vi "Define DataGrid Columns.vi"(8 "error in (no error)":errorcluster, 10 "ColumnSetup":T1[](array[typedef]) {"MinWidth" min=2 step=1; "AutoSizeMode" items=["None"=1, "ColumnHeader"=2, "AllCellsExceptHeader"=4, "AllCells"=6, "DisplayedCellsExceptHeader"=8, "DisplayedCells"=10, "Fill"=16]; "FillWeight" min=1 max=100}, 11 "DataGrid in":refnum<class "DataGridView.lvclass">) -> (0 "error out":errorcluster, 2 "ColumnDefs":refnum<class "GridColumn.lvclass">[](array[class]), 3 "DataGrid out":refnum<class "DataGridView.lvclass">)   [LabVIEW 2016, in "DataGrid.lvlib" / "DataGridView.lvclass"]
doc: "Defines the columns of the dataTable that is used to store all display data. If called more than once, it will add columns to the existing dataTable, so resulting in more (possibly duplicate) columns."
uses:
  <userlib>/LabVIEWdotNetDataGrid/source/DataGridView/DataGridView.lvclass
  <userlib>/LabVIEWdotNetDataGrid/source/GridColumn/ColumnDefinition.ctl
  <userlib>/LabVIEWdotNetDataGrid/source/GridColumn/ColumnType.ctl
  <userlib>/LabVIEWdotNetDataGrid/source/GridColumn/GridColumn.lvclass
  <userlib>/LabVIEWdotNetDataGrid/source/DataGridView/DataGridView.lvclass/DataGridView.ctl
  System.Windows.Forms
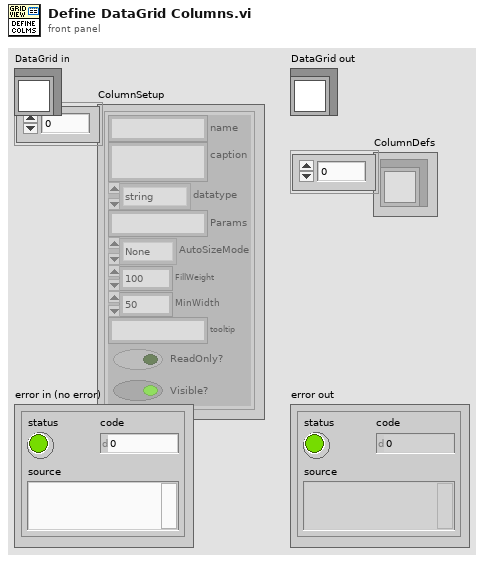
[diagram p1: front panel]
types:
  T1 = typedef "DataGrid.lvlib/GridColumn.lvclass/ColumnDefinition.ctl" = cluster{"name":string, "caption":string, "datatype":T2, "Params":string, "AutoSizeMode":i32, "FillWeight":sgl, "MinWidth":u32, "tooltip":string, "ReadOnly?":bool, "Visible?":bool}
  T2 = typedef "DataGrid.lvlib/GridColumn.lvclass/ColumnType.ctl" = enum16{"string", "image", "check", "numeric", "timestamp", "button", "combo", "link"}
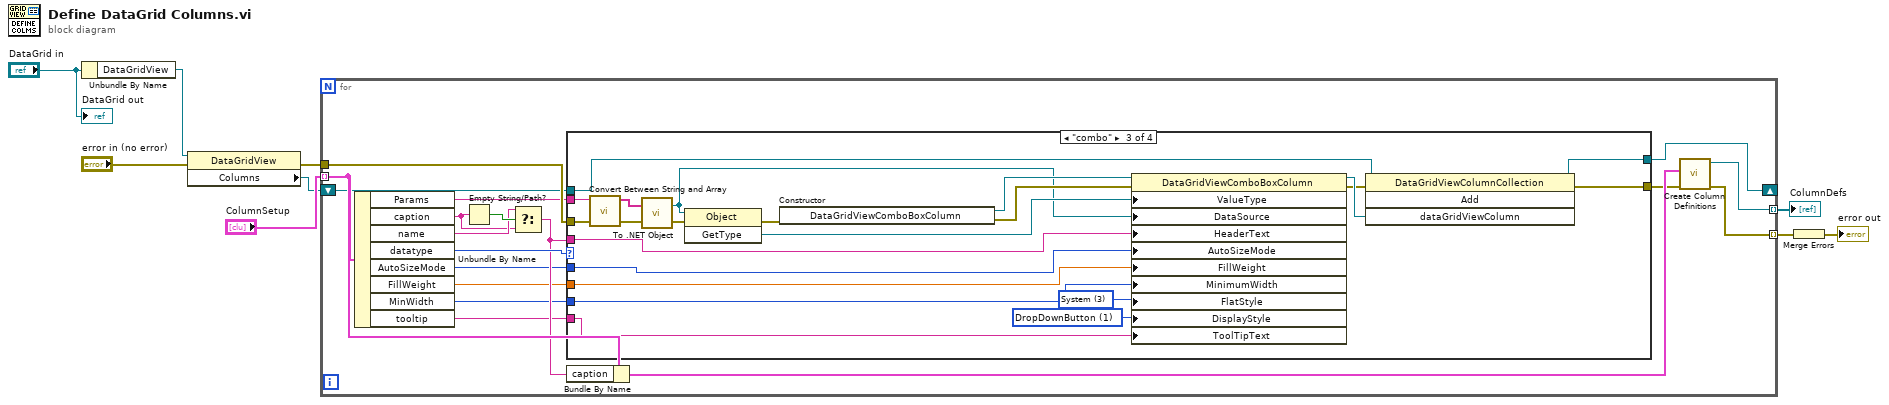
[diagram p0: block diagram]
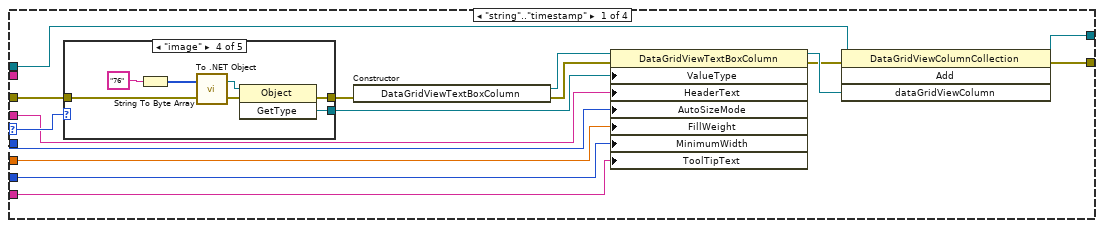
[diagram p2: hidden frame]
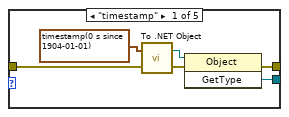
[diagram p3: hidden frame]
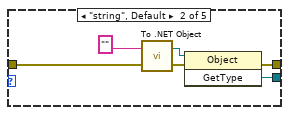
[diagram p4: hidden frame]
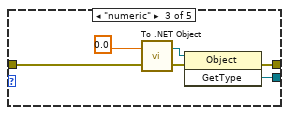
[diagram p5: hidden frame]
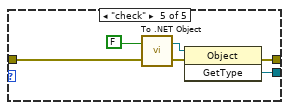
[diagram p6: hidden frame]
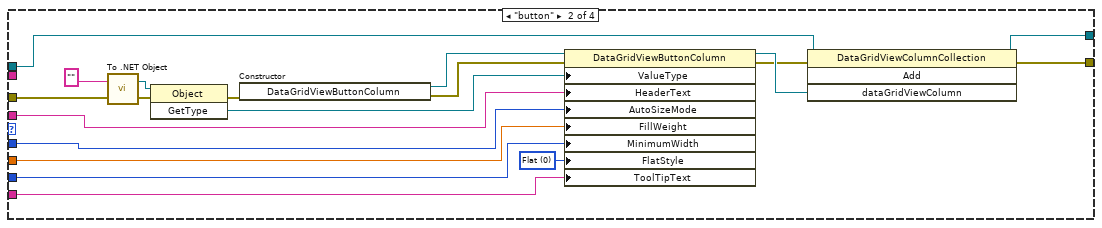
[diagram p7: hidden frame]
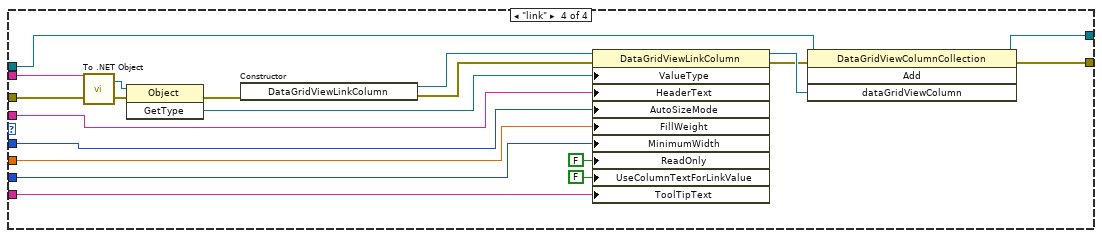
[diagram p8: hidden frame]
diagram:
  n1 = Unbundle By Name("DataGrid in") -> ("DataGridView"=w4:refnum<k24>)
  n2 = property class="DataGridView"(reference=w4, error in="error in (no error)") -> (error out=w2:errorcluster, "Columns"=w5:refnum<k24>)  [unwired: 1 out]
  n3 = for {
    tunnel: "ColumnSetup" -> [w22] mode=indexing
    tunnel: [w12] -> w7 mode=indexing
    shift-right: [w13] -> _
    shift-left: w5 -> [w14]
    tunnel: [w26] -> w6 mode=indexing
    tunnel: w2 -> [w25]
    n4 = Unbundle By Name(w22) -> ("Params"=w11:string, "caption"=w20:string, "name"=w23:string, "datatype"=w27:T2, "AutoSizeMode"=w16:i32, "FillWeight"=w17:sgl, "MinWidth"=w18:u32, "tooltip"=w10:string)
    n5 = Empty String/Path?(string/path=w20) -> (empty?=w24:bool)
    n6 = Select(t=w23, s=w24, f=w20) -> (s? t:f=w19:string)
    n7 = case shown="\"combo\"" w27 {
      selector: w27 -> [w35 _ _ _]
      tunnel: [w32 w79 w103 w122] -> w15
      tunnel: w25 -> [w43 w93 w114 w134]
      tunnel: w19 -> [w30 w76 w100 w119]
      tunnel: w18 -> [w42 w92 w113 w133]
      tunnel: w17 -> [w41 w91 w112 w132]
      tunnel: w16 -> [w40 w90 w111 w131]
      tunnel: w14 -> [w29 w78 w102 w121]
      tunnel: [w31 w77 w101 w120] -> w13
      tunnel: w11 -> [_ _ w99 w116]
      tunnel: w10 -> [w28 w75 w94 w115]
      frame "string".."timestamp" {
        n8 = case shown="\"image\"" w35 {
          tunnel: w43 -> [w47 w53 w59 w66 w72]
          tunnel: [w46 w52 w58 w65 w71] -> w38
          tunnel: [w45 w51 w57 w64 w70] -> w36
          frame "timestamp" {
            n9 = call <vilib>:"To .NET Object.vi"("error in (no error)"=w47, "anything"=timestamp(0 s since 1904-01-01) ("name")) -> ("error out"=w48:errorcluster, ".NET object"=w49:refnum<k24>)
            n10 = invoke class="Object" method="GetType"(reference=w49, error in=w48) -> (error out=w45:errorcluster, "GetType"=w46:refnum<k24>)  [unwired: 1 in, 1 out]
          }
          frame "string", Default {
            n11 = call <vilib>:"To .NET Object.vi"("error in (no error)"=w53, "anything"="") -> ("error out"=w54:errorcluster, ".NET object"=w55:refnum<k24>)
            n12 = invoke class="Object" method="GetType"(reference=w55, error in=w54) -> (error out=w51:errorcluster, "GetType"=w52:refnum<k24>)  [unwired: 1 in, 1 out]
          }
          frame "numeric" {
            n13 = call <vilib>:"To .NET Object.vi"("error in (no error)"=w59, "anything"=0.0) -> ("error out"=w60:errorcluster, ".NET object"=w61:refnum<k24>)
            n14 = invoke class="Object" method="GetType"(reference=w61, error in=w60) -> (error out=w57:errorcluster, "GetType"=w58:refnum<k24>)  [unwired: 1 in, 1 out]
          }
          frame "image" {
            n15 = String To Byte Array(string="76") -> (unsigned byte array=w62:u8[])
            n16 = call <vilib>:"To .NET Object.vi"("error in (no error)"=w66, "anything"=w62) -> ("error out"=w67:errorcluster, ".NET object"=w68:refnum<k24>)
            n17 = invoke class="Object" method="GetType"(reference=w68, error in=w67) -> (error out=w64:errorcluster, "GetType"=w65:refnum<k24>)  [unwired: 1 in, 1 out]
          }
          frame "check" {
            n18 = call <vilib>:"To .NET Object.vi"("error in (no error)"=w72, "anything"=FALSE) -> ("error out"=w73:errorcluster, ".NET object"=w74:refnum<k24>)
            n19 = invoke class="Object" method="GetType"(reference=w74, error in=w73) -> (error out=w70:errorcluster, "GetType"=w71:refnum<k24>)  [unwired: 1 in, 1 out]
          }
        }
        n20 = constructor class="DataGridViewTextBoxColumn"(error in=w36) -> (reference out=w39:refnum<k24>, error out=w37:errorcluster)  [unwired: 2 in, 1 out]
        n21 = property class="DataGridViewTextBoxColumn"(reference=w39, error in=w37, "ValueType"=w38, "HeaderText"=w30, "AutoSizeMode"=w40, "FillWeight"=w41, "MinimumWidth"=w42, "ToolTipText"=w28) -> (reference out=w34:refnum<k24>, error out=w33:errorcluster)
        n22 = invoke class="DataGridViewColumnCollection" method="Add"(reference=w29, error in=w33, "dataGridViewColumn"=w34) -> (reference out=w31:refnum<k24>, error out=w32:errorcluster)  [unwired: 1 in, 2 out]
      }
      frame "button" {
        w82 = 0 items=["Flat", "Popup", "Standard", "System"] ("FlatStyle")
        n23 = call <vilib>:"To .NET Object.vi"("error in (no error)"=w93, "anything"="") -> ("error out"=w85:errorcluster, ".NET object"=w86:refnum<k24>)
        n24 = invoke class="Object" method="GetType"(reference=w86, error in=w85) -> (error out=w88:errorcluster, "GetType"=w89:refnum<k24>)  [unwired: 1 in, 1 out]
        n25 = constructor class="DataGridViewButtonColumn"(error in=w88) -> (reference out=w83:refnum<k24>, error out=w87:errorcluster)  [unwired: 2 in, 1 out]
        n26 = property class="DataGridViewButtonColumn"(reference=w83, error in=w87, "ValueType"=w89, "HeaderText"=w76, "AutoSizeMode"=w90, "FillWeight"=w91, "MinimumWidth"=w92, "FlatStyle"=w82, "ToolTipText"=w75) -> (reference out=w81:refnum<k24>, error out=w80:errorcluster)
        n27 = invoke class="DataGridViewColumnCollection" method="Add"(reference=w78, error in=w80, "dataGridViewColumn"=w81) -> (reference out=w77:refnum<k24>, error out=w79:errorcluster)  [unwired: 1 in, 2 out]
      }
      frame "combo" {
        w97 = 1 items=["ComboBox", "DropDownButton", "Nothing"] ("DisplayStyle")
        w106 = 3 items=["Flat", "Popup", "Standard", "System"] ("FlatStyle")
        n28 = call <userlib>:"Convert Between String and Array.vi"("String"=w99) -> ("String Array"=w98:string[])  [unwired: 9 in, 1 out]
        n29 = call <vilib>:"To .NET Object.vi"("error in (no error)"=w114, "anything"=w98) -> ("error out"=w108:errorcluster, ".NET object"=w95:refnum<k24>)
        n30 = invoke class="Object" method="GetType"(reference=w95, error in=w108) -> (error out=w110:errorcluster, "GetType"=w96:refnum<k24>)  [unwired: 1 in, 1 out]
        n31 = constructor class="DataGridViewComboBoxColumn"(error in=w110) -> (reference out=w107:refnum<k24>, error out=w109:errorcluster)  [unwired: 2 in, 1 out]
        n32 = property class="DataGridViewComboBoxColumn"(reference=w107, error in=w109, "ValueType"=w96, "DataSource"=w95, "HeaderText"=w100, "AutoSizeMode"=w111, "FillWeight"=w112, "MinimumWidth"=w113, "FlatStyle"=w106, "DisplayStyle"=w97, "ToolTipText"=w94) -> (reference out=w105:refnum<k24>, error out=w104:errorcluster)
        n33 = invoke class="DataGridViewColumnCollection" method="Add"(reference=w102, error in=w104, "dataGridViewColumn"=w105) -> (reference out=w101:refnum<k24>, error out=w103:errorcluster)  [unwired: 1 in, 2 out]
      }
      frame "link" {
        n34 = call <vilib>:"To .NET Object.vi"("error in (no error)"=w134, "anything"=w116) -> ("error out"=w126:errorcluster, ".NET object"=w127:refnum<k24>)
        n35 = invoke class="Object" method="GetType"(reference=w127, error in=w126) -> (error out=w129:errorcluster, "GetType"=w130:refnum<k24>)  [unwired: 1 in, 1 out]
        n36 = constructor class="DataGridViewLinkColumn"(error in=w129) -> (reference out=w125:refnum<k24>, error out=w128:errorcluster)  [unwired: 2 in, 1 out]
        n37 = property class="DataGridViewLinkColumn"(reference=w125, error in=w128, "ValueType"=w130, "HeaderText"=w119, "AutoSizeMode"=w131, "FillWeight"=w132, "MinimumWidth"=w133, "ReadOnly"=FALSE, "UseColumnTextForLinkValue"=FALSE, "ToolTipText"=w115) -> (reference out=w124:refnum<k24>, error out=w123:errorcluster)
        n38 = invoke class="DataGridViewColumnCollection" method="Add"(reference=w121, error in=w123, "dataGridViewColumn"=w124) -> (reference out=w120:refnum<k24>, error out=w122:errorcluster)  [unwired: 1 in, 2 out]
      }
    }
    n39 = Bundle By Name(cluster=w22, "caption"=w19) -> (w21:T1)
    n40 = call <userlib>:"Create Column Definitions.vi"("error in (no error)"=w15, "Column"=w21) -> ("error out"=w12:errorcluster, "GridColumn out"=w26:refnum<class "GridColumn.lvclass">)  [unwired: 8 in]
  }
  "ColumnDefs" <- w6
  n41 = Merge Errors(w7) -> (→"error out":errorcluster)
  "DataGrid out" <- "DataGrid in"
